vi "release entry.vi"(8 "error in (no error)":errorcluster, 11 "id":string) -> (0 "error out":errorcluster)   [LabVIEW 2024, in "status manager.lvlib"]
uses:
  status manager.lvlib
  logger actions.ctl
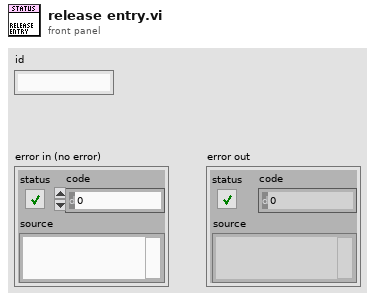
[diagram p1: front panel]
types:
  T1 = typedef "status manager.lvlib/logger actions.ctl" = enum16{"insert", "remove"}
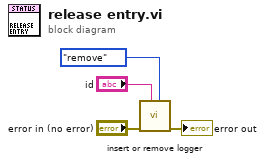
[diagram p0: block diagram]
diagram:
  n1 = call "insert or remove logger.vi"("action"=logger_actions."remove", "handler name"="id", "error in (no error)"="error in (no error)") -> ("error out"=→"error out":errorcluster)  [unwired: 8 in]
